vi "Producto Seleccionado.vi"(8 "error in":errorcluster, 9 "Costo":dbl, 10 "Unidades":i32, 11 "Nombre Producto":string) -> (0 "error out":errorcluster)   [LabVIEW 2024, in "ProductControl.lvlib"]
doc: "_____\nCreated using DQMH Framework: Event Scripter 7.1.1.1528."
uses:
  ProductControl.lvlib
  Producto Seleccionado Argument--cluster.ctl
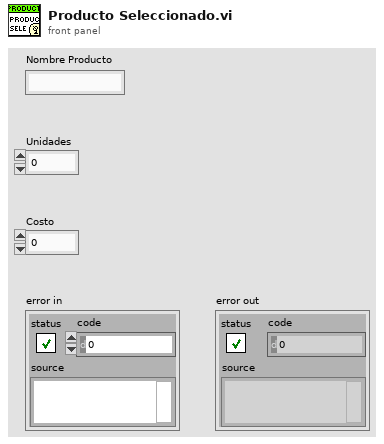
[diagram p1: front panel]
types:
  T1 = typedef "ProductControl.lvlib/Producto Seleccionado Argument--cluster.ctl" = cluster{"Nombre Producto":string, "Unidades":i32, "Costo":dbl}
  T2 = typedef "ProductControl.lvlib/Broadcast Events--cluster.ctl" = cluster{"Module Did Init":refnum<user-event>, "Status Updated":refnum<user-event>, "Error Reported":refnum<user-event>, "Module Did Stop":refnum<user-event>, "Update Module Execution Status":refnum<user-event>, "Producto Seleccionado":refnum<user-event>}
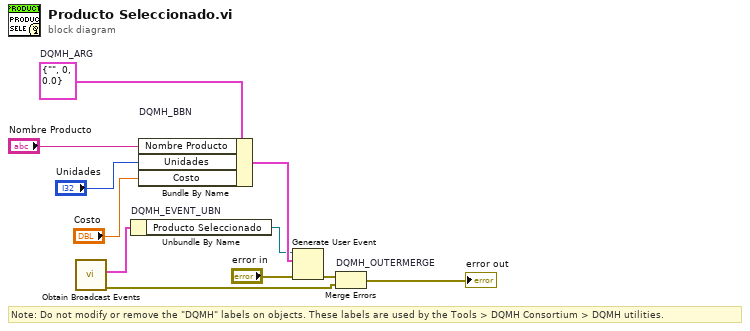
[diagram p0: block diagram]
diagram:
  w6 = T1 {"Nombre Producto"="", "Unidades"=0, "Costo"=0.0}  # DQMH_ARG
  # "Note: Do not modify or remove the \"DQMH\" labels on objects. These labels are used by the Tools > DQMH Consortium > DQMH utilities."
  n1 = call "Obtain Broadcast Events.vi"() -> ("error out"=w2:errorcluster, "ProductControl Broadcast Events"=w1:T2)  [unwired: 10 in]
  n2 = Unbundle By Name "DQMH_EVENT_UBN"(w1) -> ("Producto Seleccionado"=w8:refnum<user-event>)
  n3 = Bundle By Name "DQMH_BBN"(cluster=w6, "Nombre Producto"="Nombre Producto", "Unidades"="Unidades", "Costo"="Costo") -> (w9:T1)
  n4 = Generate User Event(user event=w8, event data cluster=w9, error in="error in") -> (error out=w7:errorcluster)  [unwired: 1 in, 1 out]
  n5 = Merge Errors "DQMH_OUTERMERGE"(w7, w2) -> (→"error out":errorcluster)
